vi "Loadfulltrackdrawing_171213.vi"(6 "Slide in 2":refnum<vi>, 8 "NormalMouseBackgroundInput":picture, 9 "BackgroundSegmentsInput":picture, 10 "360Y":dbl[](array[numeric]), 11 "360X":dbl[](array[numeric])) -> (1 "HeatMap":dbl[][](graph), 2 "NormalMousebackgroundOutput":picture, 3 "BackgroundSegmentsOutput":picture)   [LabVIEW 2016]
panel:
  in  "BinSize":i32=4
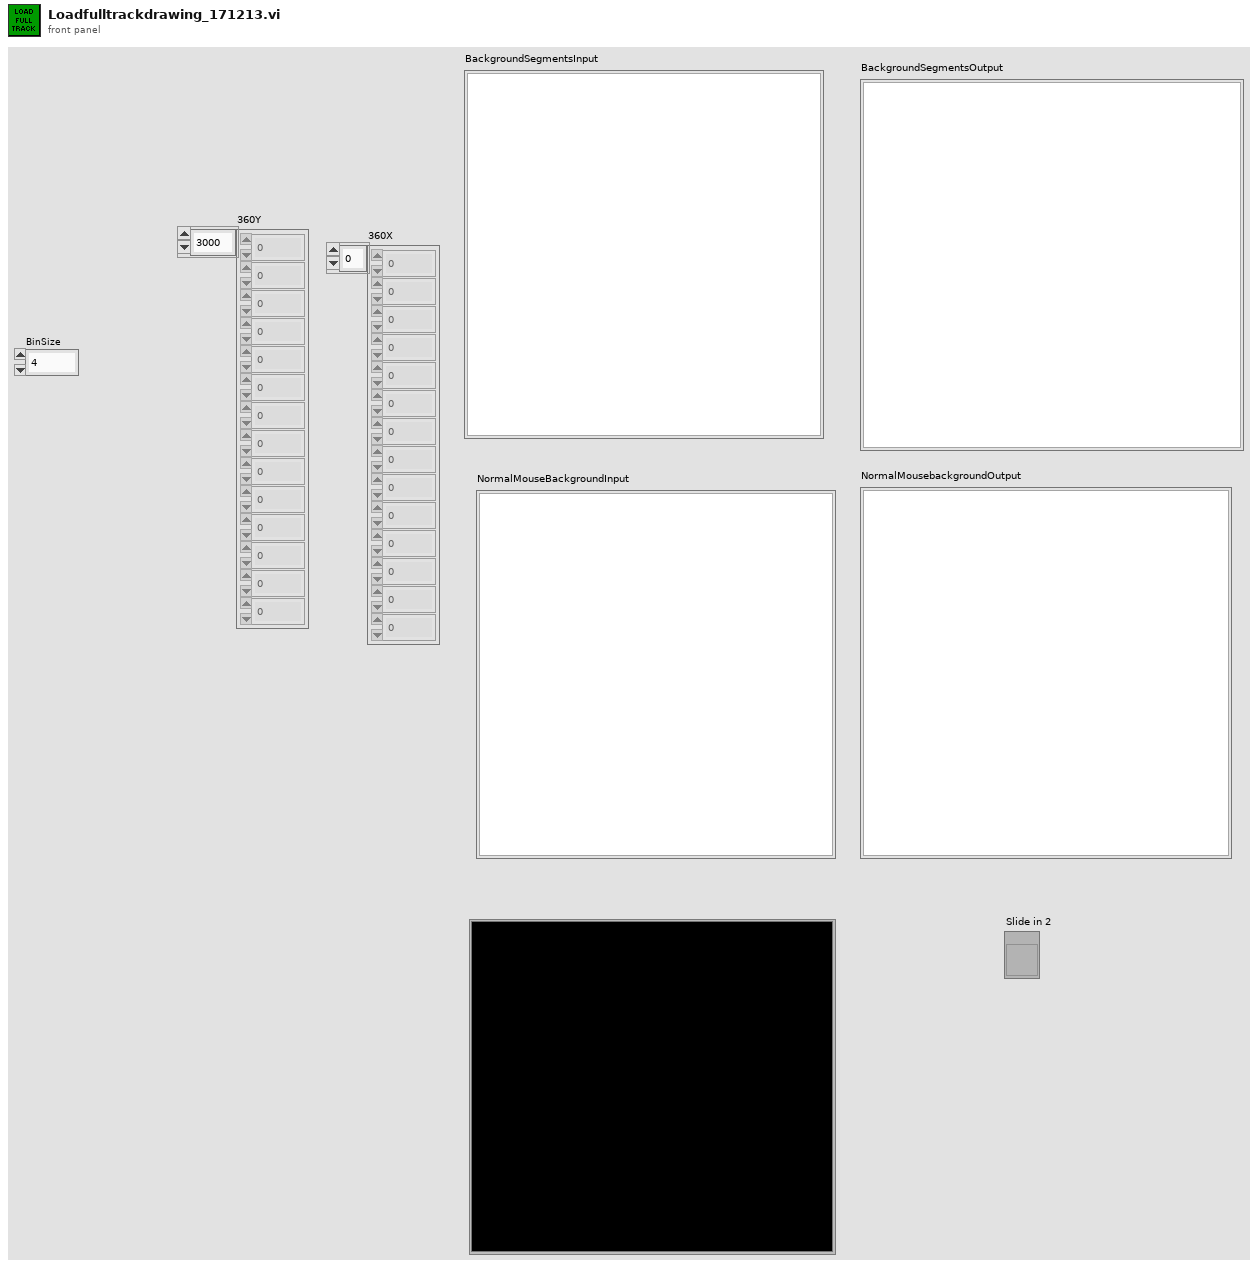
[diagram p1: front panel]
types:
  T1 = cluster{"Width":u16, "Style":enum32{"Solid", "Dash", "Dot", "DashDot", "DashDotDot"}}
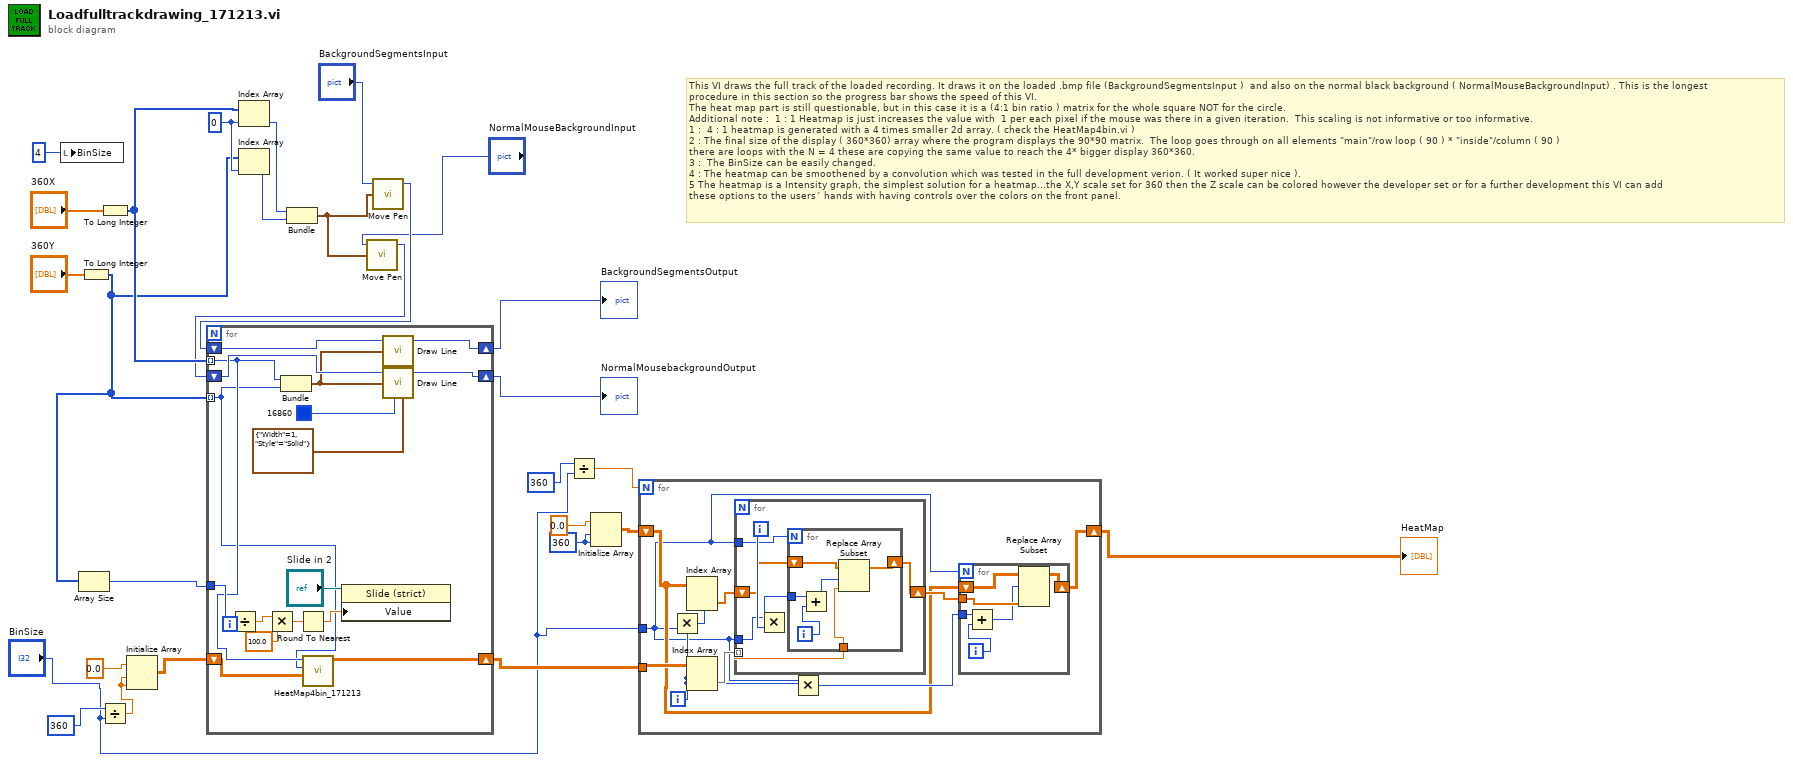
[diagram p0: block diagram]
diagram:
  w14 = 360 ("dimension size")
  w27 = 0 ("index")
  # "This VI draws the full track of the loaded recording. It draws it on the loaded .bmp file (BackgroundSegmentsInput )  and also on the normal black background ( NormalMouseBackgroundInput) . This is the longest\nprocedure in this section so the progress bar shows the speed of this VI. \nThe heat map part is still questionable, but in this case it is a (4:1 bin ratio ) matrix for the whole square NOT for the circle.\nAdditional note :  1 : 1 Heatmap is just increases the value with  1 per each pixel if the mouse was there in a given iteration.  This scaling is not informative or too informative.\n1 :  4 : 1 heatmap is generated with a 4 times smaller 2d array. ( check the HeatMap4bin.vi )\n2 : The final size of the display ( 360*360) array where the program displays the 90*90 matrix.  The loop goes through on all elements \"main\"/row loop ( 90 ) * \"inside\"/column ( 90 )\nthere are loops with the N = 4 these are copying the same value to reach the 4* bigger display 360*360.  \n3 :  The BinSize can be easily changed. \n4 : The heatmap can be smoothened by a convolution which was tested in the full development verion. ( It worked super nice ).  \n5 The heatmap is a Intensity graph, the simplest solution for a heatmap...the X,Y scale set for 360 then the Z scale can be colored however the developer set or for a further development this VI can add \nthese options to the users´ hands with having controls over the colors on the front panel."
  n1 = local write "BinSize"(4 ("BinSize")) -> ()
  n2 = To Long Integer(number="360Y") -> (32bit integer=w19:i32[])
  n3 = Array Size(array=w19) -> (size(s)=w18:i32)
  n4 = To Long Integer(number="360X") -> (32bit integer=w25:i32[])
  n5 = Divide(x=360, y="BinSize") -> (x/y=w5:dbl)
  n6 = Initialize Array(0.0 ("element"), w5, w5) -> (w16:dbl[][])
  n7 = Index Array(array=w25, index=w27) -> (element=w22:i32)
  n8 = Index Array(array=w19, index=w27) -> (element=w21:i32)
  n9 = Bundle(w22, w21) -> (w20:cluster{i32, i32})  [unwired: 1 in]
  n10 = call <vilib>:"Move Pen.vi"("new position"=w20, "picture"="NormalMouseBackgroundInput") -> ("new picture"=w23:picture)  [unwired: 3 in]
  n11 = call <vilib>:"Move Pen.vi"("new position"=w20, "picture"="BackgroundSegmentsInput") -> ("new picture"=w24:picture)  [unwired: 3 in]
  n12 = for {
    tunnel: w25 -> [w30] mode=indexing
    tunnel: w19 -> [w29] mode=indexing
    shift-right: [w45] -> w7
    shift-left: w24 -> [w46]
    shift-right: [w43] -> w10
    shift-left: w23 -> [w44]
    tunnel: w18 -> [w38]
    shift-right: [w31] -> w12
    shift-left: w16 -> [w32]
    i -> [w39]
    w42 = T1 {"Width"=1, "Style"=enum."Solid"} ("pen")
    w41 = u32 16860 ("color(black)")
    n13 = Divide(x=w39, y=w38) -> (x/y=w37:dbl)
    n14 = Multiply(x=w37, y=100.0) -> (x*y=w35:dbl)
    n15 = Bundle(w30, w29) -> (w40:cluster{i32, i32})  [unwired: 1 in]
    n16 = Round To Nearest(number=w35) -> (nearest integer value=w33:dbl)
    n17 = call "HeatMap4bin_171213.vi"("Array in"=w32, "Y"=w29, "X"=w30) -> ("Array out"=w31:dbl[][])  [unwired: 8 in]
    n18 = property class="Slide (strict)"(reference="Slide in 2", "Value"=w33) -> ()  [unwired: 1 in, 2 out]
    n19 = call <vilib>:"Draw Line.vi"("picture"=w46, "end point"=w40, "color(black)"=w41, "pen"=w42) -> ("new picture"=w45:picture)  [unwired: 5 in]
    n20 = call <vilib>:"Draw Line.vi"("picture"=w44, "end point"=w40, "color(black)"=w41, "pen"=w42) -> ("new picture"=w43:picture)  [unwired: 5 in]
  }
  "BackgroundSegmentsOutput" <- w7
  "NormalMousebackgroundOutput" <- w10
  n21 = Divide(x=360, y="BinSize") -> (x/y=w3:dbl)
  n22 = Initialize Array(0.0 ("element"), w14, w14) -> (w15:dbl[][])
  n23 = for {
    N: w3 -> [_]
    tunnel: w12 -> [w54]
    shift-right: [w48] -> w11
    shift-left: w15 -> [w49]
    tunnel: "BinSize" -> [w47]
    i -> [w52]
    n24 = Multiply(x=w52, y=w47) -> (x*y=w53:i32)
    n25 = Index Array(array=w49, index (row)=w53) -> (element=w56:dbl[])  [unwired: 1 in]
    n26 = Index Array(array=w54, index (row)=w52) -> (element=w55:dbl[])  [unwired: 1 in]
    n27 = for {
      tunnel: w55 -> [w61] mode=indexing
      shift-right: [w59] -> w50
      shift-left: w56 -> [w60]
      tunnel: w47 -> [w58]
      tunnel: w47 -> [w57]
      i -> [w62]
      n28 = Multiply(x=w58, y=w62) -> (x*y=w63:i32)
      n29 = for {
        N: w57 -> [_]
        shift-right: [w66] -> w59
        shift-left: w60 -> [w67]
        tunnel: w63 -> [w65]
        tunnel: w61 -> [w64]
        i -> [w68]
        n30 = Add(x=w65, y=w68) -> (x+y=w69:i32)
        n31 = Replace Array Subset(array=w67, new element=w64, index=w69) -> (w66:dbl[])
      }
    }
    n32 = Multiply(x=w47, y=w52) -> (x*y=w51:i32)
    n33 = for {
      N: w47 -> [_]
      shift-right: [w74] -> w48
      shift-left: w49 -> [w75]
      tunnel: w50 -> [w73]
      tunnel: w51 -> [w70]
      i -> [w72]
      n34 = Add(x=w70, y=w72) -> (x+y=w71:i32)
      n35 = Replace Array Subset(array=w75, new element=w73, index (row)=w71) -> (w74:dbl[][])  [unwired: 1 in]
    }
  }
  "HeatMap" <- w11
